vi "20SimModelSettings.vi"(10 "Set finish time":dbl=-1.0) -> (0 "period_ms":i32, 1 "OutputsArray":dbl[](array[numeric]), 2 "finishtime":dbl, 3 "starttime":dbl, 4 "stepsize":dbl, 5 "InputsArray":dbl[](array[numeric]), 6 "outputs":i32, 7 "inputs":i32)   [LabVIEW 2011]
uses:
  lv20simmodel.dll
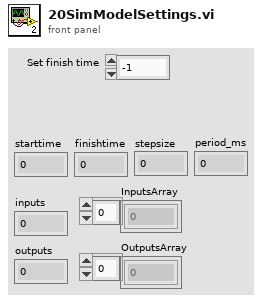
[diagram p1: front panel]
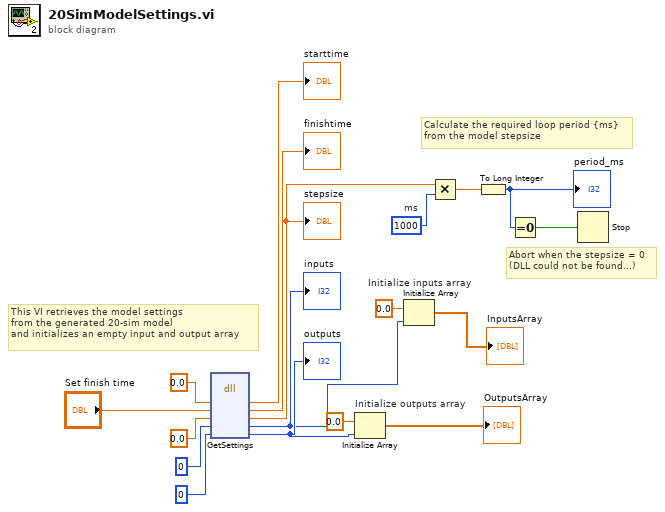
[diagram p0: block diagram]
diagram:
  w5 = 1000  # ms
  # "Calculate the required loop period {ms}\nfrom the model stepsize"
  # "Abort when the stepsize = 0\n(DLL could not be found...)"
  # "This VI retrieves the model settings\nfrom the generated 20-sim model\nand initializes an empty input and output array"
  n1 = dll-call lib="C:/Temp/BondGraphModel/lv20simmodel.dll" fn="GetSettings"("starttime"=0.0, "finishtime"="Set finish time", "stepsize"=0.0, "inputs"=0, "outputs"=0) -> ("starttime"=→"starttime":dbl, "finishtime"=→"finishtime":dbl, "stepsize"=w2:dbl, "inputs"=w8:i32, "outputs"=w15:i32)  [unwired: 4 in, 2 out]
  "stepsize" <- w2
  "outputs" <- w15
  "inputs" <- w8
  n2 = Initialize Array "Initialize outputs array"(0.0, w15) -> (→"OutputsArray":dbl[])
  n3 = Initialize Array "Initialize inputs array"(0.0, w8) -> (→"InputsArray":dbl[])
  n4 = Multiply(x=w2, y=w5) -> (x*y=w4:dbl)
  n5 = To Long Integer(number=w4) -> (32bit integer=w1:i32)
  "period_ms" <- w1
  n6 = Equal To 0?(x=w1) -> (x = 0?=w3:bool)
  n7 = Stop(stop? (T)=w3) -> ()
